vi "acqInitLasersFW.vi"(2 "LSFM_3 lasers":T1(array[cluster])=[{"Component ID"="405nm", "COM Port"="COM14", "Type "=enum."omicronLuxX", "init"=0, "Max power (mW)"=60.0}, {"Component ID"="488nm", "COM Port"="COM4", "Type "=enum."omicronLuxX", "init"=0, "Max power (mW)"=60.0}, {"Component ID"="561nm", "COM Port"="COM27", "Type "=enum."coherentObis", "init"=0, "Max power (mW)"=50.0}, {"Component ID"="642nm", "COM Port"="COM12", "Type "=enum."omicronLuxX", "init"=0, "Max power (mW)"=140.0}], 6 "405 nm (aq)":bool=TRUE, 7 "405 filter":u8(ring)=1 items=["460/36 [DAPI]"=1, "525/50 [FITC]"=2, "605/70 [Cy3]"=3, "665/LP [Cy5]"=4, "Empty-1"=5, "Empty-2"=6], 8 "488 nm (aq)":bool=TRUE, 9 "488 filter":u8(ring)=2 items=["460/36 [DAPI]"=1, "525/50 [FITC]"=2, "605/70 [Cy3]"=3, "665/LP [Cy5]"=4, "Empty-1"=5, "Empty-2"=6], 10 "561 nm (aq)":bool=TRUE, 11 "561 filter":u8(ring)=3 items=["460/36 [DAPI]"=1, "525/50 [FITC]"=2, "605/70 [Cy3]"=3, "665/LP [Cy5]"=4, "Empty-1"=5, "Empty-2"=6], 12 "642 nm (aq)":bool=TRUE, 13 "642 filter":u8(ring)=4 items=["460/36 [DAPI]"=1, "525/50 [FITC]"=2, "605/70 [Cy3]"=3, "665/LP [Cy5]"=4, "Empty-1"=5, "Empty-2"=6]) -> (15 "FWpos":u8[](array[numeric]), 16 "acqLaserCOM":refnum<visa-resource-name>[](array[refnum]), 17 "acqLaserOn":string[](array[string]), 18 "acqLaserOff":string[](array[string]))   [LabVIEW 2015]
panel:
  out "Correct lasers init?":i16=1
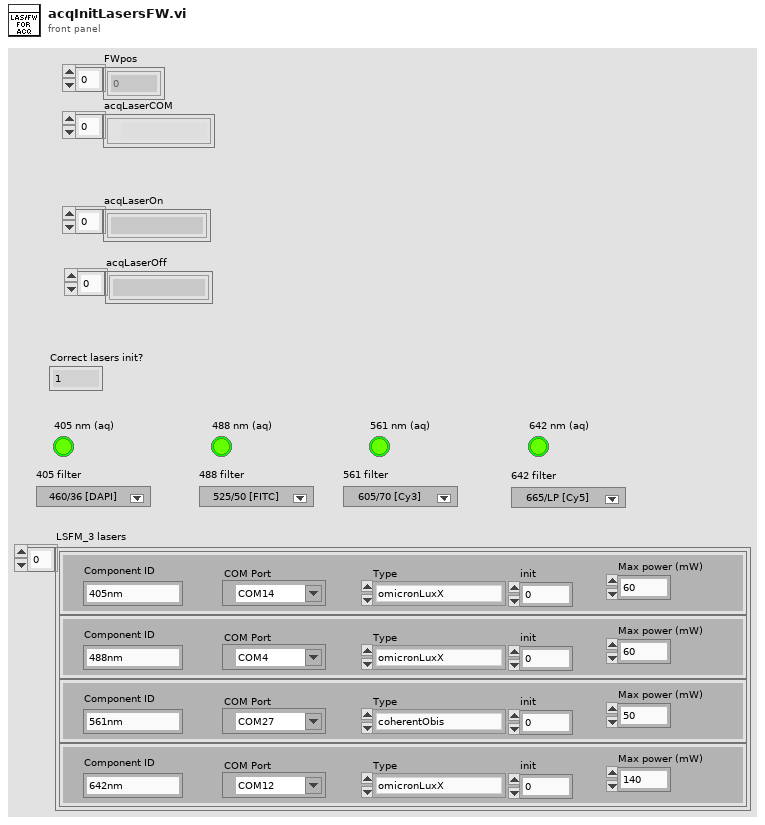
[diagram p1: front panel]
types:
  T1 = cluster{"Component ID":string, "COM Port":refnum<visa-resource-name>, "Type ":enum16{"omicronLuxX", "coherentObis"}, "init":i16, "Max power (mW)":dbl}[]
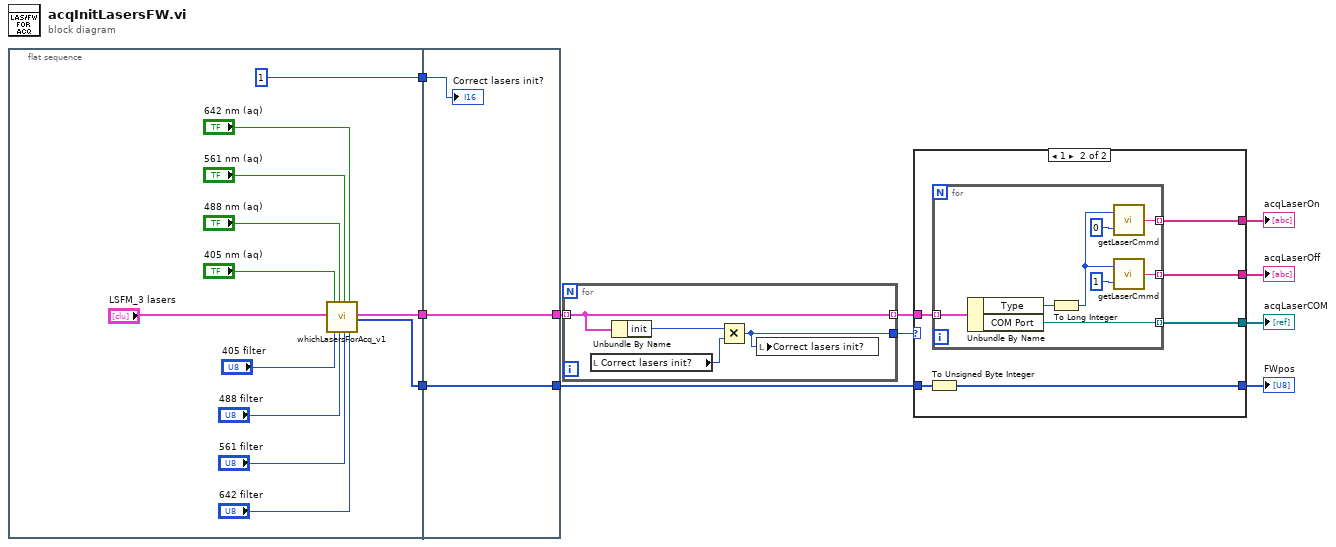
[diagram p0: block diagram]
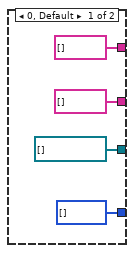
[diagram p2: hidden frame]
diagram:
  n1 = flat-sequence {
    tunnel: [w23] -> w3
    tunnel: [w22] -> w2
    tunnel: [i16 1 ("Correct lasers init?")] -> w1
    tunnel: [w25] -> w5
    tunnel: [w26] -> w7
    tunnel: w3 -> [w26]
    tunnel: w2 -> [w25]
    tunnel: w1 -> [w24]
    frame #0 {
      n2 = call "whichLasersForAcq_v1.vi"("LSFM_3 lasers"="LSFM_3 lasers", "405 nm (aq)"="405 nm (aq)", "405 filter"="405 filter", "488 nm (aq)"="488 nm (aq)", "488 filter"="488 filter", "561 nm (aq)"="561 nm (aq)", "561 filter"="561 filter", "642 nm (aq)"="642 nm (aq)", "642 filter"="642 filter") -> ("initLasers"=w22:T1, "initFilters"=w23:u8[])  [unwired: 9 in]
    }
    frame #1 {
      "Correct lasers init?" <- w24
    }
  }
  n3 = for {
    tunnel: w5 -> [w28] mode=indexing
    tunnel: [w29] -> w4
    tunnel: [w28] -> w6 mode=indexing
    n4 = local read "Correct lasers init?"() -> (w30:i16)
    n5 = Unbundle By Name(w28) -> ("init"=w27:i16)
    n6 = Multiply(x=w27, y=w30) -> (x*y=w29:i16)
    n7 = local write "Correct lasers init?"(w29) -> ()
  }
  n8 = case shown="1" w4 {
    tunnel: [string[] [] w40] -> w11
    tunnel: [string[] [] w39] -> w10
    tunnel: [refnum<visa-resource-name>[] [] w38] -> w9
    tunnel: w6 -> [_ w37]
    tunnel: w7 -> [_ w36]
    tunnel: [u8[] [] w35] -> w8
    frame 0, Default {
    }
    frame 1 {
      n9 = To Unsigned Byte Integer(number=w36) -> (unsigned 8bit integer=w35:u8[])
      n10 = for {
        tunnel: w37 -> [w48] mode=indexing
        tunnel: [w47] -> w38 mode=indexing
        tunnel: [w42] -> w40 mode=indexing
        tunnel: [w41] -> w39 mode=indexing
        n11 = Unbundle By Name(w48) -> ("Type"=w46:enum16{"omicronLuxX", "coherentObis"}, "COM Port"=w47:refnum<visa-resource-name>)
        n12 = To Long Integer(number=w46) -> (32bit integer=w45:i32)
        n13 = call "getLaserCmmd.vi"("Cmmd index"=0, "Laser type"=w45) -> ("Laser command"=w42:string)
        n14 = call "getLaserCmmd.vi"("Cmmd index"=1, "Laser type"=w45) -> ("Laser command"=w41:string)
      }
    }
  }
  "FWpos" <- w8
  "acqLaserCOM" <- w9
  "acqLaserOff" <- w10
  "acqLaserOn" <- w11
